vi "Bar1001.vi"   [LabVIEW 2013]
uses:
  <vilib>/Heliosphere Research LLC/Advanced Plotting Toolkit/Advanced Plotting Toolkit.lvlib
types:
  T1 = typedef "Advanced Plotting Toolkit.lvlib/PlotID.ctl" = i32
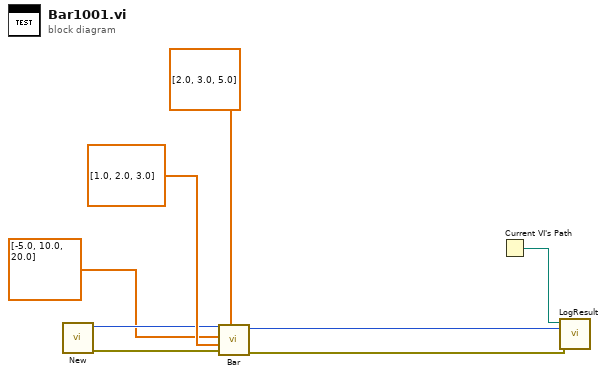
[diagram p0: block diagram]
diagram:
  n1 = call <vilib>:"New.vi"() -> ("error out"=w4:errorcluster, "Plot ID"=w6:T1)  [unwired: 10 in]
  n2 = call <vilib>:"Bar.vi"("Bar Widths"=dbl[] [2.0, 3.0, 5.0], "error in (no error)"=w4, "Bar Lengths"=dbl[] [1.0, 2.0, 3.0], "X Coordinates"=dbl[] [-5.0, 10.0, 20.0], "Plot ID"=w6) -> ("error out"=w3:errorcluster, "Plot ID Out"=w5:T1)  [unwired: 5 in]
  n3 = Current VI's Path() -> (path=w8:path)
  n4 = call "LogResult.vi"("Test Result"=w3, "Test Artifact"=w5, "VI Path"=w8) -> ()  [unwired: 9 in]
